vi "Activity_11.vi"() -> ()   [LabVIEW 2015]
panel:
  out "Parking lot":bool[][](array[boolean])=[[FALSE, FALSE, FALSE, FALSE, FALSE, FALSE, FALSE, FALSE, FALSE, FALSE, FALSE], [FALSE, FALSE, FALSE, FALSE, FALSE, FALSE, FALSE, FALSE, FALSE, FALSE, FALSE], [FALSE, FALSE, FALSE, FALSE, FALSE, FALSE, FALSE, FALSE, FALSE, FALSE, FALSE], [FALSE, FALSE, FALSE, FALSE, FALSE, FALSE, FALSE, FALSE, FALSE, FALSE, FALSE], [FALSE, FALSE, FALSE, FALSE, FALSE, FALSE, FALSE, FALSE, FALSE, FALSE, FALSE], [FALSE, FALSE, FALSE, FALSE, FALSE, FALSE, FALSE, FALSE, FALSE, FALSE, FALSE], [FALSE, FALSE, FALSE, FALSE, FALSE, FALSE, FALSE, FALSE, FALSE, FALSE, FALSE], [FALSE, FALSE, FALSE, FALSE, FALSE, FALSE, FALSE, FALSE, FALSE, FALSE, FALSE], [FALSE, FALSE, FALSE, FALSE, FALSE, FALSE, FALSE, FALSE, TRUE, FALSE, FALSE], [FALSE, FALSE, FALSE, FALSE, FALSE, FALSE, FALSE, FALSE, FALSE, FALSE, FALSE]]
  in  "stop":bool
  in  "Columns\nsize":i32=10
  in  "Rows\nsize":i32=10
  # "Serrano Bermúdez Luis Esteban"
  # "Simulador de un Estacionamiento"
  # "Fecha de Entrega: 23/Febrero/2019"
  # "Simula la entrada de automoviles en un arreglo de LEDS\nde manera aleatoria.\nLa cantidad de filas y columnas se puede elegir por medio\nde los controles \"Rows Size\" y \"Column Size\""
  # "Descripción:"
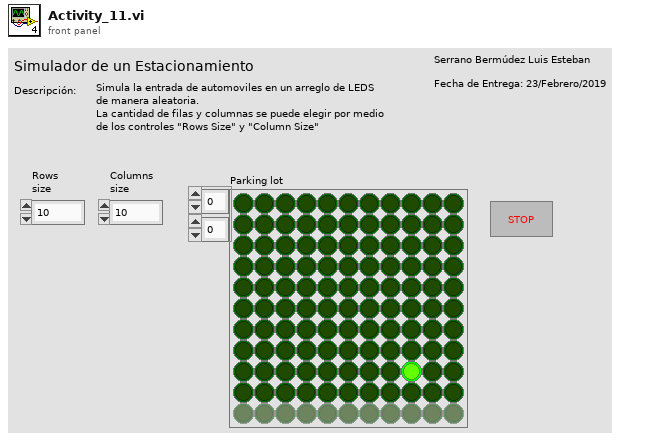
[diagram p1: front panel]
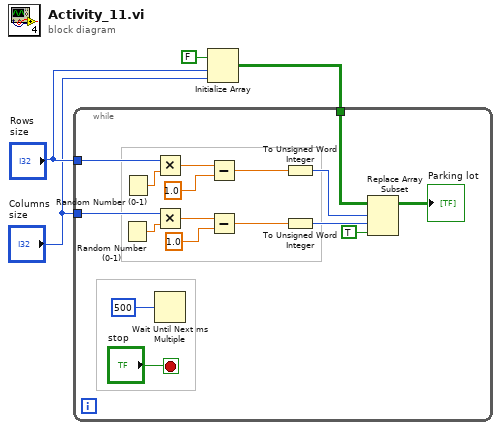
[diagram p0: block diagram]
diagram:
  n1 = Initialize Array(FALSE, "Rows\nsize", "Columns\nsize") -> (w1:bool[][])
  n2 = while {
    tunnel: "Rows\nsize" -> [w11]
    tunnel: "Columns\nsize" -> [w10]
    tunnel: w1 -> [w7]
    stop <- "stop" stop-if-true
    n3 = Random Number (0-1)() -> (number: 0 to 1=w13:dbl)
    n4 = Random Number (0-1)() -> (number: 0 to 1=w14:dbl)
    n5 = Multiply(x=w11, y=w14) -> (x*y=w19:dbl)
    n6 = Multiply(x=w10, y=w13) -> (x*y=w16:dbl)
    n7 = Wait Until Next ms Multiple(millisecond multiple=u32 500) -> ()  [unwired: 1 out]
    n8 = Subtract(x=w19, y=1.0) -> (x-y=w18:dbl)
    n9 = Subtract(x=w16, y=1.0) -> (x-y=w17:dbl)
    n10 = To Unsigned Word Integer(number=w18) -> (unsigned 16bit integer=w6:u16)
    n11 = To Unsigned Word Integer(number=w17) -> (unsigned 16bit integer=w5:u16)
    n12 = Replace Array Subset(array=w7, new element=TRUE ("new element/subarray"), index (row)=w6, index (col)=w5) -> (→"Parking lot":bool[][])
  }
